vi "Horizontal Splitter.vi"(6 "Splitter Position":i32, 8 "error in (no error)":errorcluster, 10 "Limits":cluster{"Left":i16, "Right":i16}) -> (0 "error out":errorcluster)   [LabVIEW 2013, in "Interaction Splitter.lvclass"]
doc: "Copyright 2018, Wiebe Walstra, wiebe@carya.nl."
uses:
  Interaction Splitter.lvclass
  <vilib>/Utility/miscctls.llb/LVPointTypeDef.ctl
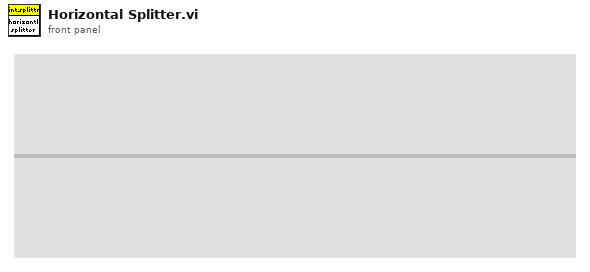
[diagram p1: front panel]
types:
  T1 = typedef "LVPointTypeDef.ctl" = cluster{"Horizontal":i16, "Vertical":i16}
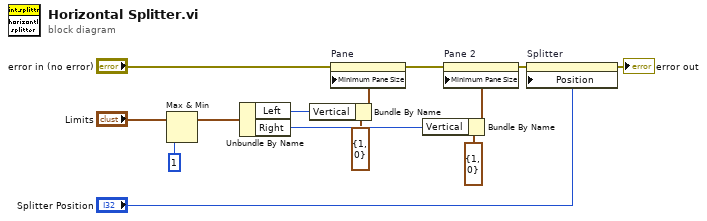
[diagram p0: block diagram]
diagram:
  n1 = Max & Min(x="Limits", y=i16 1 ("Horizontal")) -> (max(x,y)=w5:cluster{"Left":i16, "Right":i16})  [unwired: 1 out]
  n2 = Unbundle By Name(w5) -> ("Left"=w9:i16, "Right"=w13:i16)
  n3 = Bundle By Name(cluster=T1 {"Horizontal"=1, "Vertical"=0} ("Minimum Pane Size"), "Vertical"=w9) -> (w8:T1)
  n4 = property on="Pane" class="Pane"(error in="error in (no error)", "Minimum Pane Size"=w8) -> (error out=w12:errorcluster)  [unwired: 1 in, 1 out]
  n5 = Bundle By Name(cluster=T1 {"Horizontal"=1, "Vertical"=0} ("Minimum Pane Size"), "Vertical"=w13) -> (w10:T1)
  n6 = property on="Pane 2" class="Pane"(error in=w12, "Minimum Pane Size"=w10) -> (error out=w2:errorcluster)  [unwired: 1 in, 1 out]
  n7 = property on="Splitter" class="Splitter"(error in=w2, "Position"="Splitter Position") -> (error out=→"error out":errorcluster)  [unwired: 1 in, 1 out]
